vi "Check Loop Error.vi"(6 "Component":string, 8 "Ignored Errors":i32[](array[numeric]), 9 "Critical Errors":i32[](array[numeric]), 10 "Error to Handle":errorcluster, 11 "Message Queue":refnum<queue>) -> ()   [LabVIEW 2024]
doc: "Determines whether an error is a critical error, non-critical error, or ignored error. If an error is a critical error or non-critical error, this VI sends an error message to the message Handling loop to handle this error."
uses:
  Support/Shared/Message Queue/Message Cluster.ctl
  Error Type.ctl
  Error Message.ctl
  Support/Shared/Message Queue.lvlib
panel:
  out "error out":errorcluster
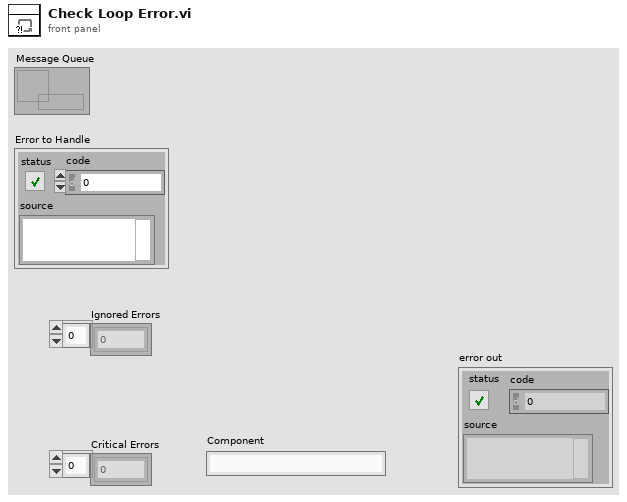
[diagram p1: front panel]
types:
  T1 = typedef "Error Message.ctl" = cluster{"Error":errorcluster, "Component":string}
  T2 = typedef "Error Type.ctl" = enum16{"Ignored Error", "Non-Critical Error", "Critical Error"}
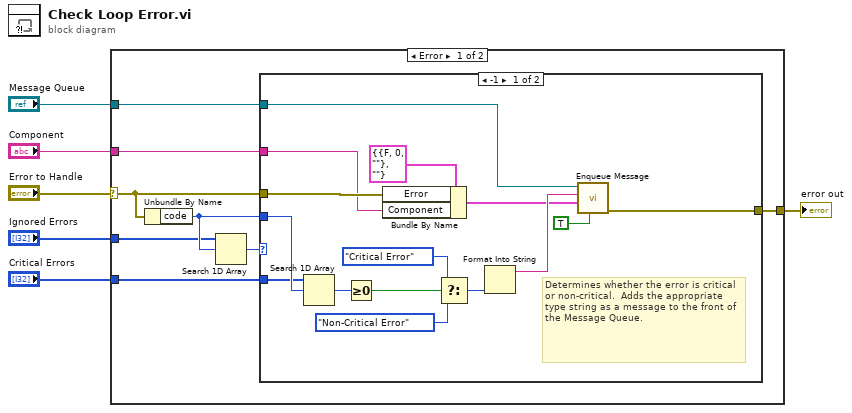
[diagram p0: block diagram]
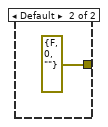
[diagram p2: hidden frame]
diagram:
  n1 = case shown="Error" "Error to Handle" {
    selector: "Error to Handle" -> [w11 w31]
    tunnel: "Message Queue" -> [w14 _]
    tunnel: "Ignored Errors" -> [w10 _]
    tunnel: "Critical Errors" -> [w9 _]
    tunnel: [w8 w31] -> w2
    tunnel: "Component" -> [w7 _]
    frame Error {
      n2 = Unbundle By Name(w11) -> ("code"=w12:i32)
      n3 = Search 1D Array(1D array=w10, element=w12) -> (index of element=w13:i32)  [unwired: 1 in]
      n4 = case shown="-1" w13 {
        tunnel: w11 -> [w23 _]
        tunnel: w14 -> [w18 _]
        tunnel: w12 -> [w29 _]
        tunnel: w9 -> [w25 _]
        tunnel: [w17 errorcluster {"status"=FALSE, "code"=0, "source"=""} ("error out")] -> w8
        tunnel: w7 -> [w16 _]
        frame -1 {
          # "Determines whether the error is critical or non-critical.  Adds the appropriate type string as a message to the front of the Message Queue."
          n5 = Search 1D Array(1D array=w25, element=w29) -> (index of element=w28:i32)  [unwired: 1 in]
          n6 = Greater Or Equal To 0?(x=w28) -> (x >= 0?=w27:bool)
          n7 = Bundle By Name(cluster=T1 {"Error"={"status"=FALSE, "code"=0, "source"=""}, "Component"=""} ("Error Message"), "Error"=w23, "Component"=w16) -> (w19:T1)
          n8 = Select(t=Error_Type."Critical Error" ("Error Type (Non-Critical)"), s=w27, f=Error_Type."Non-Critical Error" ("Error Type (Non-Critical)")) -> (s? t:f=w20:T2)
          n9 = Format Into String(w20) -> (resulting string=w21:string)  [unwired: 3 in, 1 out]
          n10 = call "Enqueue Message.vi"("Priority Message? (F)"=TRUE, "Message Data"=w19, "Message"=w21, "Message Queue"=w18) -> ("error out"=w17:errorcluster)  [unwired: 6 in, 1 out]
        }
        frame Default {
        }
      }
    }
    frame No Error {
    }
  }
  "error out" <- w2
